vi "Download Last Stock Price.vi"(8 "error in (no error)":errorcluster caption="entrée d'erreur (pas d'erreur)", 11 "Share en entrée":refnum<class "Stock.lvclass"> caption="DNL_LabVIEW Object in") -> (0 "error out":errorcluster caption="sortie d'erreur", 1 "Last Price":dbl, 2 "Download OK":bool, 3 "Share en sortie":refnum<class "Stock.lvclass"> caption="DNL_LabVIEW Object out")   [LabVIEW 2012, in "Stock.lvclass"]
uses:
  Stock.lvclass
  Stock.lvclass/Stock.ctl
  <vilib>/httpClient/LabVIEWHTTPClient.lvlib
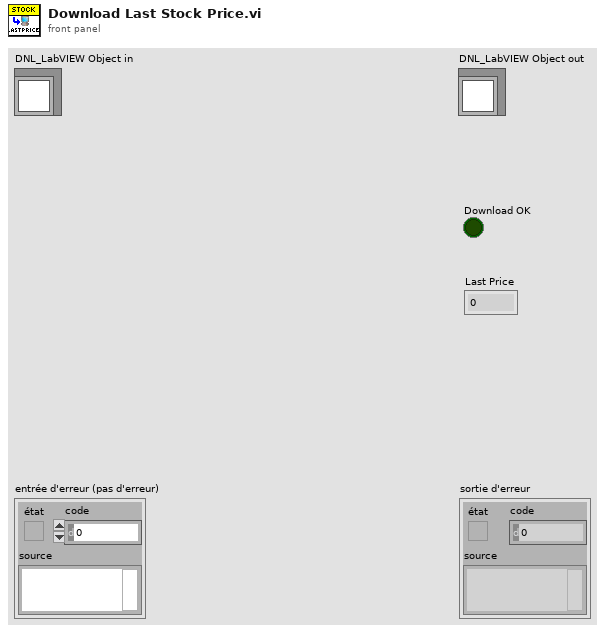
[diagram p1: front panel]
types:
  T1 = typedef "LabVIEWHTTPClient.lvlib/ClientHandle.ctl" = refnum<k1>
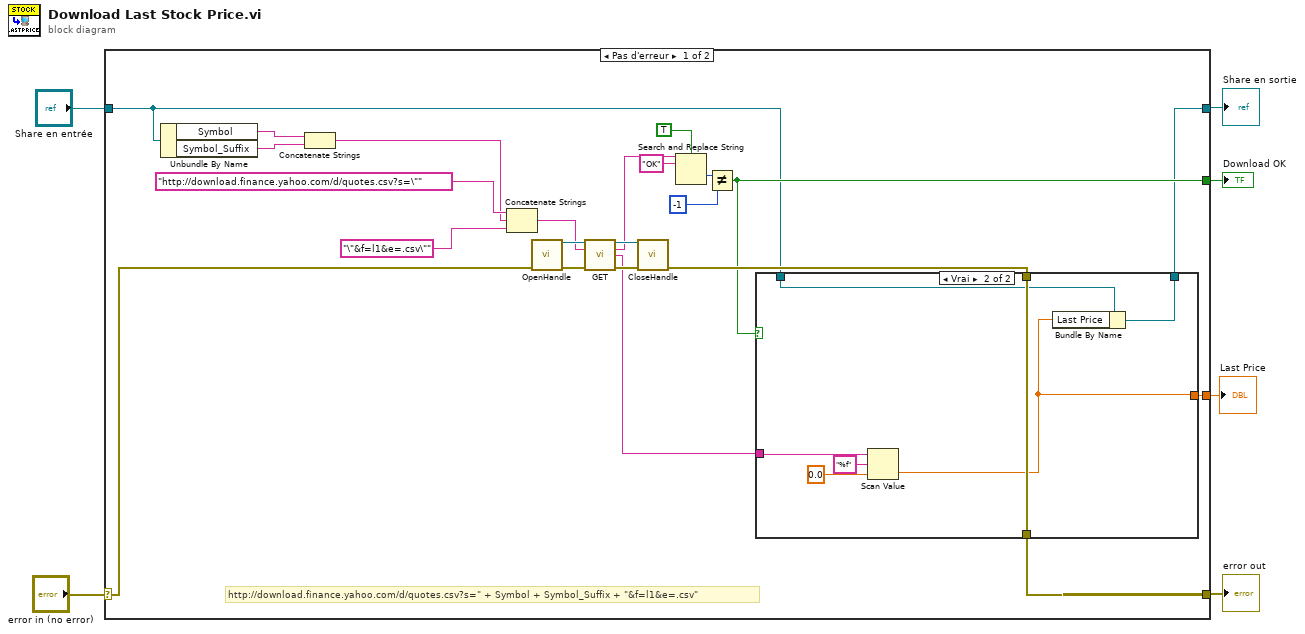
[diagram p0: block diagram]
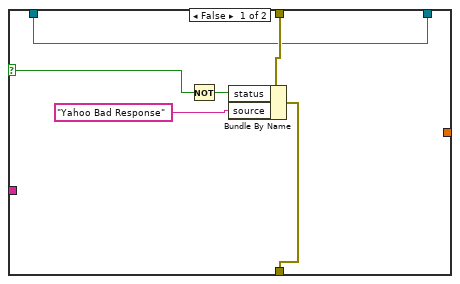
[diagram p2: hidden frame]
diagram:
  n1 = case shown="Pas d'erreur" "error in (no error)" {
    selector: "error in (no error)" -> [w22 w44]
    tunnel: [w11 w44] -> w5
    tunnel: [w8 w43] -> w3
    tunnel: "Share en entrée" -> [w9 w43]
    tunnel: [w12 _] -> w2
    tunnel: [w7 _] -> w1
    frame No Error {
      # "http://download.finance.yahoo.com/d/quotes.csv?s=\" + Symbol + Symbol_Suffix + \"&f=l1&e=.csv\""
      n2 = Unbundle By Name(w9) -> ("Symbol"=w29:string, "Symbol_Suffix"=w28:string)
      n3 = Concatenate Strings(w29, w28) -> (w13:string)
      n4 = Concatenate Strings("http://download.finance.yahoo.com/d/quotes.csv?s=\"", w13, "\"&f=l1&e=.csv\"") -> (w24:string)
      n5 = call <vilib>:"OpenHandle.vi"("error in (no error)"=w22) -> ("client handle out"=w27:T1, "error out"=w21:errorcluster)  [unwired: 13 in]
      n6 = call <vilib>:"GET.vi"("client handle"=w27, "url"=w24, "error in (no error)"=w21) -> ("client handle out"=w23:T1, "headers"=w19:string, "body"=w10:string, "error out"=w20:errorcluster)  [unwired: 9 in]
      n7 = call <vilib>:"CloseHandle.vi"("client handle"=w23, "error in (no error)"=w20) -> ("error out"=w14:errorcluster)  [unwired: 13 in]
      n8 = Search and Replace String(case sensitive?=TRUE ("ignorer la casse ? (F)"), input string=w19, search string="OK" ("chaîne recherchée")) -> (offset past replacement=w16:i32)  [unwired: 5 in, 3 out]
      n9 = Not Equal?(x=w16, y=-1) -> (x != y?=w12:bool)
      n10 = case shown="Vrai" w12 {
        selector: w12 -> [w33 _]
        tunnel: w14 -> [w35 w42]
        tunnel: [w34 w42] -> w11
        tunnel: w10 -> [_ w38]
        tunnel: w9 -> [w30 w41]
        tunnel: [w30 w40] -> w8
        tunnel: [_ w36] -> w7
        frame False {
          n11 = Not(x=w33) -> (.not. x?=w32:bool)
          n12 = Bundle By Name(cluster=w35, "status"=w32, "source"="Yahoo Bad Response" ("chaîne recherchée")) -> (w34:errorcluster)
        }
        frame True {
          n13 = Scan Value(string=w38, format string="%f" ("chaîne de format"), default (0 dbl)=0.0 ("entrée 1")) -> (value=w36:dbl)  [unwired: 1 out]
          n14 = Bundle By Name(cluster=w41, "Last Price"=w36) -> (w40:refnum<class "Stock.lvclass">)
        }
      }
    }
    frame Error {
    }
  }
  "error out" <- w5
  "Share en sortie" <- w3
  "Download OK" <- w2
  "Last Price" <- w1
